vi "Diff IO Interface.vi"(6 "Device Inputs":dbl[](array[numeric]), 8 "error in":errorcluster, 9 "Device Outputs in":dbl[](array[numeric]), 10 "DCM Ref":refnum<class "DCM - RT.lvclass">, 11 "Diff IO in":T1={"DiffIO Command Enabled"=FALSE, "FIFO Indexes"={"Read"={"Diff IO Results"=[], "DiffIOIn"={"1"=-1, "2"=-1, "3"=-1, "4"=-1, "5"=-1, "6"=-1, "7"=-1, "8"=-1}}, "Write"={"Diff I/O Setup"=[]}}}) -> (0 "error out":errorcluster, 1 "Device Outputs out":dbl[](array[numeric]))   [LabVIEW 2016, in "DCM Engine.lvlib"]
uses:
  DCM Engine.lvlib
  Built/DCM Classes Packed/Pharlap/C/DCM-Classes.lvlibp/DCM/Rev0/RT/DCM - RT.lvclass
  Shared/Types/DiffIO.ctl
  Shared/Types/DiffIO Results Indexes.ctl
  Shared/Types/DiffIO Setup Indexes.ctl
  Built/DCM Classes Packed/Pharlap/C/DCM-Classes.lvlibp/DCM/Diff IO/RT/DCM - RT - Diff IO.lvlib
  DCM Shared.lvlib
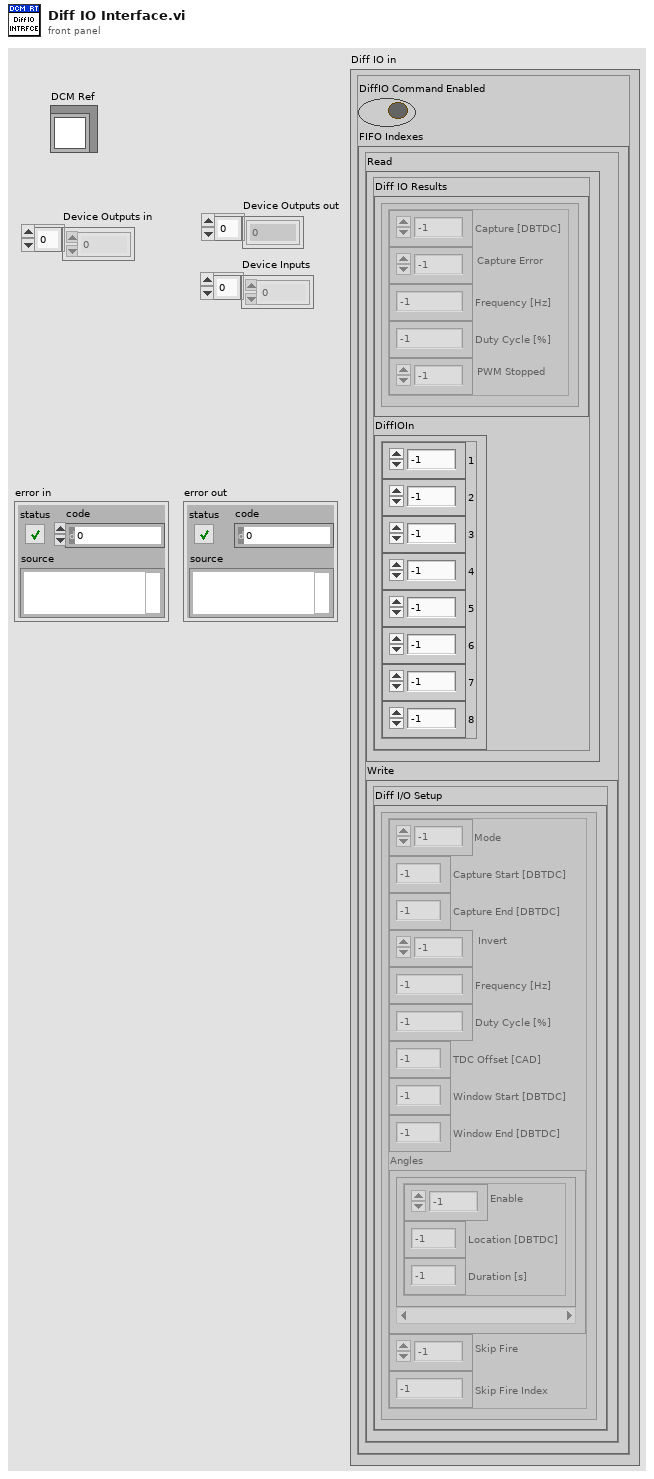
[diagram p1: front panel]
types:
  T1 = typedef "DCM Shared.lvlib/DiffIO.ctl" = cluster{"DiffIO Command Enabled":bool, "FIFO Indexes":cluster{"Read":cluster{"Diff IO Results":T2[], "DiffIOIn":cluster{"1":i32, "2":i32, "3":i32, "4":i32, "5":i32, "6":i32, "7":i32, "8":i32}}, "Write":cluster{"Diff I/O Setup":T3[]}}}
  T2 = typedef "DCM Shared.lvlib/DiffIO Results Indexes.ctl" = cluster{"Capture [DBTDC]":i32, "Capture Error":i32, "Frequency [Hz]":i32, "Duty Cycle [%]":i32, "PWM Stopped":i32}
  T3 = typedef "DCM Shared.lvlib/DiffIO Setup Indexes.ctl" = cluster{"Mode":i32, "Capture Start [DBTDC]":i32, "Capture End [DBTDC]":i32, "Invert":i32, "Frequency [Hz]":i32, "Duty Cycle [%]":i32, "TDC Offset [CAD]":i32, "Window Start [DBTDC]":i32, "Window End [DBTDC]":i32, "Angles":cluster{"Enable":i32, "Location [DBTDC]":i32, "Duration [s]":i32}[], "Skip Fire":i32, "Skip Fire Index":i32}
  T4 = cluster{"Diff IO Results":T2[], "DiffIOIn":cluster{"1":i32, "2":i32, "3":i32, "4":i32, "5":i32, "6":i32, "7":i32, "8":i32}}
  T5 = typedef "DCM-Classes.lvlibp/DCM - RT - Diff IO.lvlib/Setup.ctl" = cluster{"Mode":T6, "Capture Start [DBTDC]":sgl, "Capture End [DBTDC]":sgl, "Invert":bool, "Frequency [Hz]":sgl, "Duty Cycle [%]":sgl, "TDC Offset [CAD]":sgl, "Window Start [DBTDC]":sgl, "Window End [DBTDC]":sgl, "Angles":T7[], "Skip Fire":bool, "Skip Fire Index":u8}
  T6 = typedef "DCM-Classes.lvlibp/DCM - FPGA - Diff IO.lvlib/Mode.ctl" = enum8{"Off", "Input", "Pulse Width Modulation", "Engine Position Tracking", "Serial Out 1", "Serial Out 2", "EPTx Sync"}
  T7 = typedef "DCM-Classes.lvlibp/DCM - RT - Diff IO.lvlib/Angle Control.ctl" = cluster{"Enable":bool, "Location [DBTDC]":sgl, "Duration [s]":sgl}
  T8 = typedef "DCM-Classes.lvlibp/DCM - RT - Diff IO.lvlib/Results.ctl" = cluster{"Capture [DBTDC]":sgl, "Capture Error":bool, "Frequency [Hz]":sgl, "Duty Cycle [%]":sgl, "PWM Stopped":bool}
  T9 = typedef "DCM-Classes.lvlibp/DCM - FPGA - Tools.lvlib/8 Channels.ctl" = cluster{"1":bool, "2":bool, "3":bool, "4":bool, "5":bool, "6":bool, "7":bool, "8":bool}
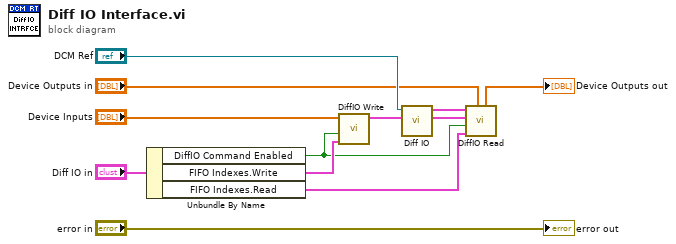
[diagram p0: block diagram]
diagram:
  n1 = Unbundle By Name("Diff IO in") -> ("DiffIO Command Enabled"=w3:bool, "FIFO Indexes.Write"=w6:cluster{"Diff I/O Setup":T3[]}, "FIFO Indexes.Read"=w4:T4)
  n2 = call "DiffIO Write.vi"("FIFO Indexes.Write"=w6, "Command Enabled"=w3, "Device Inputs"="Device Inputs") -> ("Diff IO Setup"=w5:T5[])  [unwired: 8 in]
  n3 = call "Diff IO.vi"("Diff IO Setup"=w5, "DCM Reference"="DCM Ref") -> ("Diff IO Results"=w2:T8[], "Diff IO In"=w1:T9)  [unwired: 8 in]
  n4 = call "DiffIO Read.vi"("Device Outputs in"="Device Outputs in", "FIFO Indexes.Read"=w4, "Command Enabled"=w3, "Diff IO Results"=w2, "Diff I/O In"=w1) -> ("Device Outputs out"=→"Device Outputs out":dbl[])  [unwired: 6 in]
  "error out" <- "error in"
